vi "Launch GUI.vi"(8 "error in (no error)":errorcluster, 11 "GUI Builder in":refnum<class "GUI Builder.lvclass">) -> (0 "error out":errorcluster)   [LabVIEW 2025, in "App-Builder Library.lvlib" / "GUI Builder.lvclass"]
uses:
  GUI Builder.lvclass
  GUI.vi
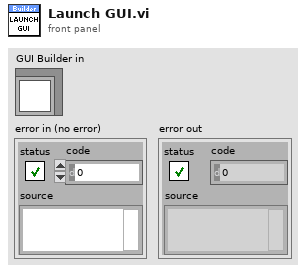
[diagram p1: front panel]
types:
  T1 = enum32{"Bad", "Idle", "Run top level", "Running"}
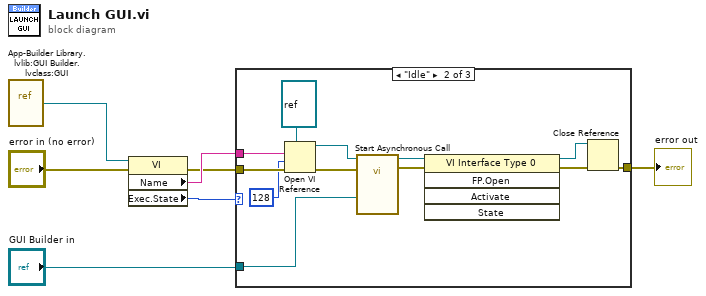
[diagram p0: block diagram]
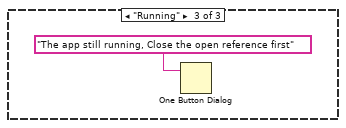
[diagram p3: hidden frame]
diagram:
  n1 = vi-ref "App-Builder Library.lvlib:GUI Builder.lvclass:GUI.vi"() -> (w7:refnum<vi>)
  n2 = property class="VI"(reference=w7, error in="error in (no error)") -> (error out=w5:errorcluster, "Name"=w6:string, "Exec.State"=w1:T1)  [unwired: 1 out]
  n3 = case shown="\"Idle\"" w1 {
    tunnel: w6 -> [_ w18 _]
    tunnel: w5 -> [_ w17 _]
    tunnel: [_ w14 _] -> w3
    tunnel: "GUI Builder in" -> [_ w13 _]
    frame Default {
    }
    frame "Idle" {
      n4 = Open VI Reference(type specifier VI Refnum (for type only)=refnum<vi> refnum, vi path=w18, options=128, error in (no error)=w17) -> (vi reference=w19:refnum<vi>, error out=w16:errorcluster)  [unwired: 2 in]
      n5 = call-by-ref "Start Asynchronous Call"(reference=w19, error in=w16, "GUI Builder in"=w13) -> (reference out=w12:refnum<vi>, error out=w9:errorcluster)  [unwired: 11 in]
      n6 = invoke class="VI Interface Type 0" method="FP.Open"(reference=w12, error in=w9) -> (reference out=w10:refnum<vi>, error out=w11:errorcluster)  [unwired: 3 in, 3 out]
      n7 = Close Reference(reference=w10, error in (no error)=w11) -> (error out=w14:errorcluster)
    }
    frame "Running" {
      n8 = One Button Dialog(message="The app still running, Close the open reference first" ("format string")) -> ()  [unwired: 1 in, 1 out]
    }
  }
  "error out" <- w3
